vi "Robot Global Data.vi"() -> ()   [LabVIEW 2012]
doc: "This global VI can contain as many global variables as you need. Place a control on the panel, give it a good name. To read or write to it from a VI, drag the icon to the diagram of that VI. You can also drag from the project. Click on the node to change which global you access. You shouldn't have multiple locations writing to a global or it will cause a race-condition."
uses:
  <vilib>/Rock Robotics/WPI/Camera/WPI_CameraImageSize.ctl
panel:
  in  "Ball scale fator":dbl
  in  "Ball Density ratio":dbl min=-10.0 max=10.0 step=0.0001
  in  "Auto":dbl=50.0
  in  "Shooter motor Speed":dbl=50.0
  in  "Key of  3 Pointer":dbl=89.0
  in  "Side of  2 Pointer 2":dbl=50.0
  in  "Frount of 2  Pointer":dbl=50.0
  in  "Frount of  3 Pointer":dbl=65.0
  in  "Angle Trim":dbl
  in  "Velocity Trim":dbl
  in  "Kinect Motor Speed":dbl=0.5
  in  "Kinect Slew Rate":dbl=0.5
  in  "Turn Table Rate":dbl=1.0
  in  "Shooter":bool
  in  "Target Distances":dbl[](array[numeric])
  in  "Ball Count":dbl
  in  "Hopper Full":bool
  out "Last Distance":dbl
  in  "Target Index":dbl
  out "Joystick Control":bool
  in  "Selected Target":i32 min=0 max=3
  out "Last Y Coordinate":dbl
  out "Y Servo Angle":dbl
  out "Last X Coordinate":dbl
  out "X Servo Angle":dbl
  out "Target Info":T1(array[cluster])
  in  "Arm Lower Limit":dbl=1.0
  in  "Arm Down Speed":dbl=-0.5
  in  "Arm Up Speed":dbl=0.5
  in  "Arm Upper Limit":dbl=1.0
  in  "Frount/Rear drive speed":dbl=0.33
  in  "MECH Rotate Speed":dbl=1.0
  in  "MECH X/Y Speed":dbl=1.0
  in  "Ball Shooter motor speed":dbl=0.5
  in  "Belt Drive Foward speed":dbl=0.5
  in  "Belt Drive Reverse speed":dbl=0.5
  in  "Sweep Drive Foward speed":dbl=0.5
  in  "Sweep Drive Reverse speed":dbl=0.5
  in  "Ball Release Delay in Milliseconds":i32=2000
  in  "Delay after Ball is Release":u32=500
  in  "Delay in Milliseconds":i32=3000
  in  "Rotation mode":enum16{"straight", "L1", "L2", "R1", "R2"}(ring)
  in  "LED toggle rate (ms)":u32=20
  in  "image size":T2=enum."320x240"
  in  "Enable Vision":bool
  # "Drive Speed"
  # "Shooter Times"
  # "Shooter Speeds"
  # "Hybrid"
  # "1000 Milliseconds = 1 Second"
  # "Shooter button"
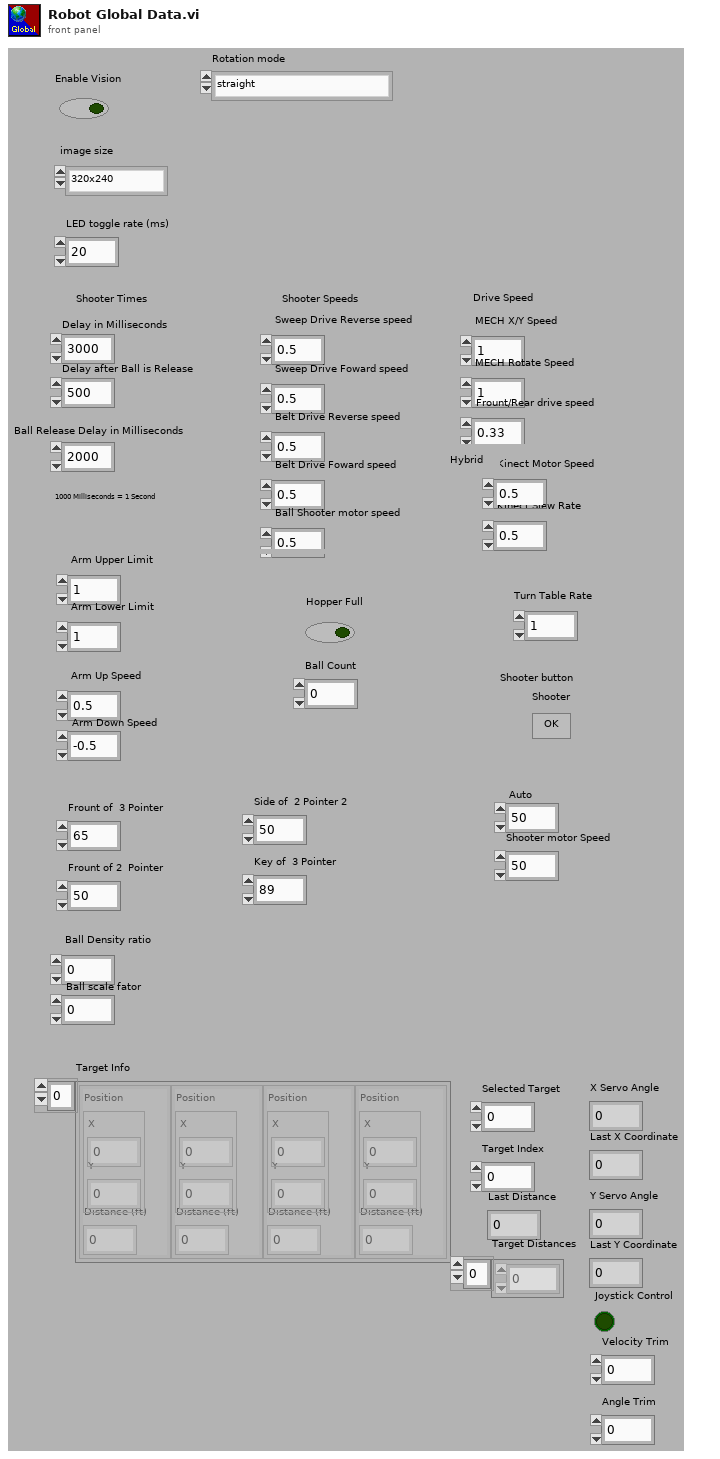
[diagram p1: front panel]
types:
  T1 = cluster{"Position":cluster{"X":dbl, "Y":dbl}, "Distance (ft)":dbl}[]
  T2 = typedef "WPI_CameraImageSize.ctl" = enum16{"640x480", "320x240", "160x120"}
diagram:
